vi "Lab01_Khongmeng_Basic_Labview.vi"() -> ()   [LabVIEW 2016]
panel:
  out "32bit integer":i32
  in  "Enum":T1(ring)
  out "small cluster 2":cluster{"Boolean 2":bool, "slide":dbl}
  out "small cluster":cluster{"Numeric":dbl, "Boolean":bool}
  in  "Cluster 2":T2 {"Slide" scale=0.0..10.0}
  out "String 4":string
  out "Numeric 2":dbl
  out "Boolean 7":bool
  out "String 3":string
  out "Company Name":string
  out "Age":dbl
  out "Employed?":bool
  out "Name":string
  in  "Cluster":T3
  in  "Input":string[](array[string])
  out "Info":string[][](array[string])
  out "Element":dbl
  out "Min":dbl
  out "Max":dbl
  out "size(s)":dbl[](array[numeric])
  out "Array 2":dbl[][](array[numeric])
  out "Array":dbl[][](array[numeric])
  out "number to string":string
  out "string to number":dbl
  in  "Info":string
  in  "Name":string
  out "formatted form":string
  out "After separation":string
  out "Before separation":string
  out "Remove him":string
  out "printf":string
  out "Boolean 5":bool
  out "Boolean 4":bool
  out "Boolean 3":bool
  in  "Boolean 2":bool
  in  "Boolean":bool
  out "|Area (cm^2)":dbl
  in  "Base (cm)":dbl
  in  "Height (cm)":dbl
  out "A-B":dbl
  out "A+B":dbl
  in  "B":dbl
  in  "A":dbl
  # "Area of  a Triangle"
  # "Height"
  # "Base"
  # "concatenate"
  # "Search & Replace"
  # "Match"
  # "Formate"
  # "row index"
  # "colomn index"
  # "Input, match, size and print"
  # "Yes"
  # "No"
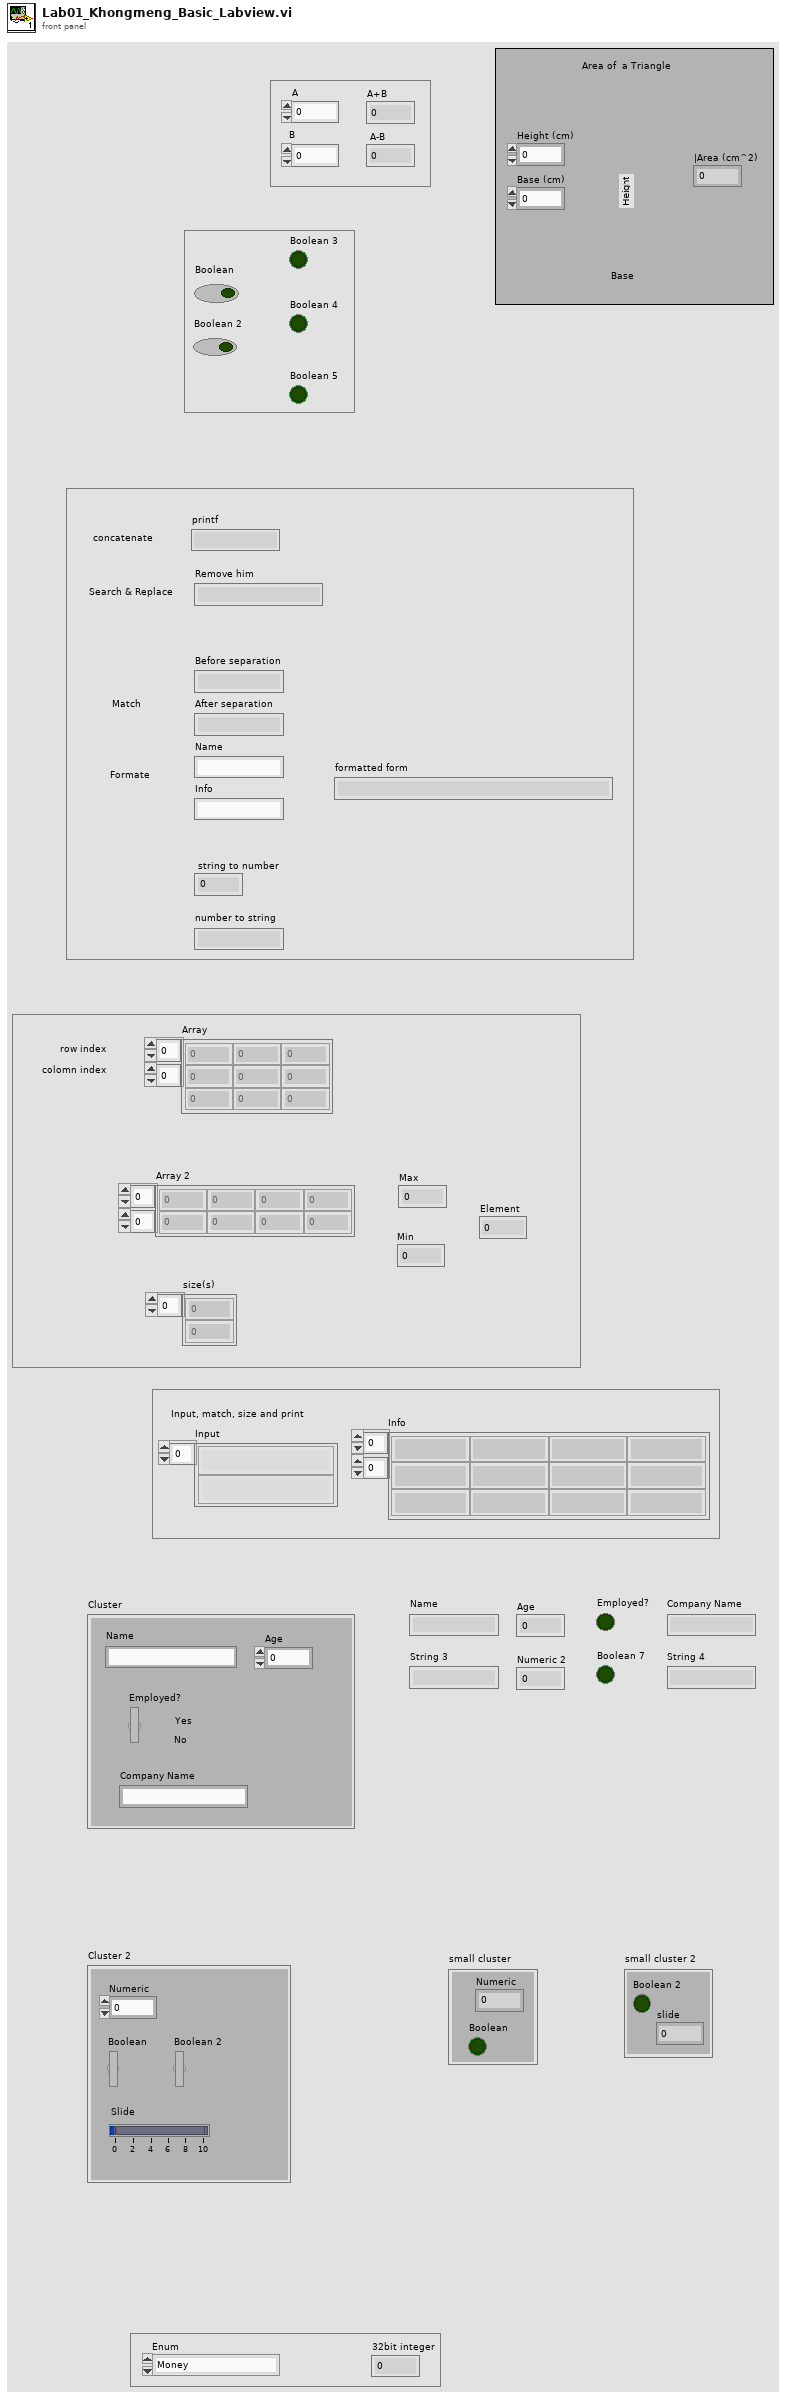
[diagram p1: front panel]
types:
  T1 = enum16{"Money", "Tuesday", "Wednesday", "Thursday", "Friday", "Saturday", "Sunday"}
  T2 = cluster{"Numeric":dbl, "Boolean":bool, "Boolean 2":bool, "Slide":dbl}
  T3 = cluster{"Name":string, "Age":dbl, "Employed?":bool, "Company Name":string}
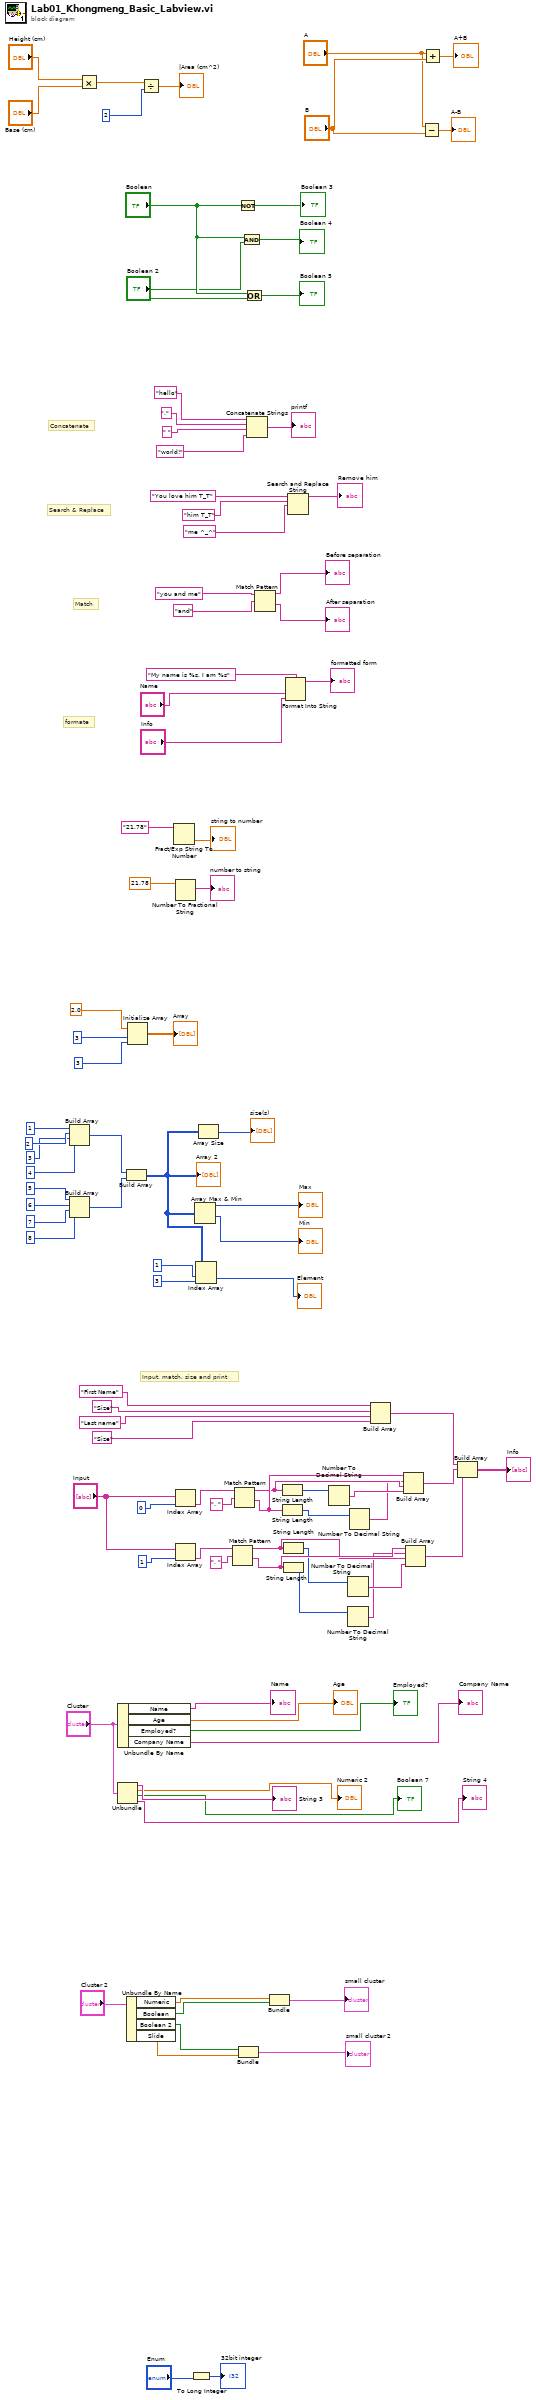
[diagram p0: block diagram]
diagram:
  # "Input, match, size and print"
  # "formate"
  # "Match"
  # "Search & Replace"
  # "Concatenate"
  n1 = Build Array(1, 2, 3, 4) -> (w54:i32[])
  n2 = Build Array(5, 6, 7, 8) -> (w53:i32[])
  n3 = Multiply(x="Height (cm)", y="Base (cm)") -> (x*y=w95:dbl)
  n4 = Unbundle("Cluster") -> ("Name"=→"String 3":string, "Age"=→"Numeric 2":dbl, "Employed?"=→"Boolean 7":bool, "Company Name"=→"String 4":string)
  n5 = Unbundle By Name("Cluster") -> ("Name"=→"Name":string, "Age"=→"Age":dbl, "Employed?"=→"Employed?":bool, "Company Name"=→"Company Name":string)
  n6 = Build Array(w54, w53) -> (w47:i32[][])
  "Array 2" <- w47
  n7 = Unbundle By Name("Cluster 2") -> ("Numeric"=w8:dbl, "Boolean"=w7:bool, "Boolean 2"=w5:bool, "Slide"=w4:dbl)
  n8 = Initialize Array(2.0, 3, 3) -> (→"Array":dbl[][])
  n9 = Divide(x=w95, y=2) -> (x/y=→"|Area (cm^2)":dbl)
  n10 = Fract/Exp String To Number(string="21,78") -> (number=→"string to number":dbl)  [unwired: 3 in, 1 out]
  n11 = Number To Fractional String(number=21.78) -> (F-format string=→"number to string":string)  [unwired: 3 in]
  n12 = Index Array(array="Input", index=0) -> (element=w38:string)
  n13 = Index Array(array="Input", index=1) -> (element=w37:string)
  n14 = To Long Integer(number="Enum") -> (32bit integer=→"32bit integer":i32)
  n15 = Array Max & Min(array=w47) -> (max value=→"Max":i32, min value=→"Min":i32)  [unwired: 2 out]
  n16 = Index Array(array=w47, index (row)=1, index (col)=3) -> (element=→"Element":i32)
  n17 = Array Size(array=w47) -> (size(s)=→"size(s)":i32[])
  n18 = Match Pattern(string=w37, regular expression=", ") -> (before substring=w31:string, after substring=w32:string)  [unwired: 1 in, 2 out]
  n19 = Match Pattern(string=w38, regular expression=", ") -> (before substring=w33:string, after substring=w34:string)  [unwired: 1 in, 2 out]
  n20 = Not(x="Boolean") -> (.not. x?=→"Boolean 3":bool)
  n21 = Bundle("Boolean 2"=w5, "Slide"=w4) -> (→"small cluster 2":cluster{"Boolean 2":bool, "Slide":dbl})  [unwired: 1 in]
  n22 = And(x="Boolean", y="Boolean 2") -> (x .and. y?=→"Boolean 4":bool)
  n23 = Or(x="Boolean", y="Boolean 2") -> (x .or. y?=→"Boolean 5":bool)
  n24 = Concatenate Strings("hello", ",", " ", "world!") -> (→"printf":string)
  n25 = Match Pattern(string="you and me", regular expression="and") -> (before substring=→"Before separation":string, after substring=→"After separation":string)  [unwired: 1 in, 2 out]
  n26 = Bundle("Numeric"=w8, "Boolean"=w7) -> (→"small cluster":cluster{"Numeric":dbl, "Boolean":bool})  [unwired: 1 in]
  n27 = String Length(string=w33) -> (length=w26:i32)
  n28 = String Length(string=w34) -> (length=w24:i32)
  n29 = String Length(string=w31) -> (length=w22:i32)
  n30 = String Length(string=w32) -> (length=w20:i32)
  n31 = Format Into String(format string="My name is %s, I am %s", "Name", "Info") -> (resulting string=→"formatted form":string)  [unwired: 2 in, 1 out]
  n32 = Search and Replace String(input string="You love him T_T", search string="him T_T", replace string="me ^_^") -> (result string=→"Remove him":string)  [unwired: 5 in, 3 out]
  n33 = Number To Decimal String(number=w26) -> (decimal integer string=w25:string)  [unwired: 1 in]
  n34 = Number To Decimal String(number=w22) -> (decimal integer string=w21:string)  [unwired: 1 in]
  n35 = Number To Decimal String(number=w20) -> (decimal integer string=w19:string)  [unwired: 1 in]
  n36 = Number To Decimal String(number=w24) -> (decimal integer string=w23:string)  [unwired: 1 in]
  n37 = Build Array("First Name", "Size", "Last name", "Size") -> (w30:string[])
  n38 = Build Array(w34, w23, w33, w25) -> (w29:string[])
  n39 = Build Array(w32, w19, w31, w21) -> (w28:string[])
  n40 = Subtract(x="A", y="B") -> (x-y=→"A-B":dbl)
  n41 = Add(x="A", y="B") -> (x+y=→"A+B":dbl)
  n42 = Build Array(w30, w29, w28) -> (→"Info":string[][])
